vi "Param_OCVACIR.vi"(8 "errin":errorcluster, 9 "section":string="Hioki BT3562", 10 "Chaîne":string, 11 "pathin":path) -> (0 "Errout":errorcluster caption="errout", 2 "DATA":T1)   [LabVIEW 2020]
uses:
  <vilib>/Utility/config.llb/Read Key (U32).vi
  <vilib>/Utility/config.llb/Read Key (Double).vi
  <vilib>/Utility/config.llb/NI_LVConfig.lvlib
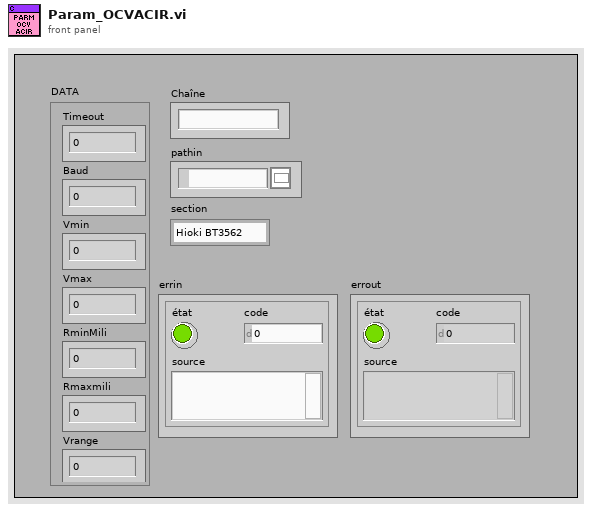
[diagram p1: front panel]
types:
  T1 = cluster{"Timeout":dbl, "Baud":u32, "Vmin":dbl, "Vmax":dbl, "RminMili":dbl, "Rmaxmili":dbl, "Vrange":dbl}
  T2 = typedef "NI_LVConfig.lvlib/Config Data RefNum.ctl" = refnum<k1>
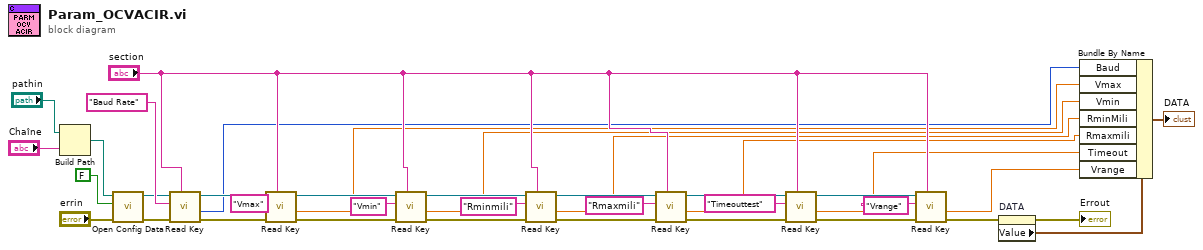
[diagram p0: block diagram]
diagram:
  n1 = Build Path(base path="pathin", name or relative path="Chaîne") -> (appended path=w18:path)
  n2 = call <vilib>:"Open Config Data.vi"("error in (no error)"="errin", "create file if necessary (T)"=FALSE, "configuration file path"=w18) -> ("error out"=w21:errorcluster, "refnum"=w17:T2)  [unwired: 6 in, 1 out]
  n3 = call-poly <vilib>:"Read Key.vi"("section"="section", "error in (no error)"=w21, "key"="Baud Rate", "refnum"=w17) -> ("error out"=w32:errorcluster, "value"=w1:u32, "refnum out"=w22:T2)  [unwired: 4 in, 1 out]
  n4 = call-poly <vilib>:"Read Key.vi"("section"="section", "error in (no error)"=w32, "key"="Vmax", "refnum"=w22) -> ("error out"=w33:errorcluster, "value"=w2:dbl, "refnum out"=w23:T2)  [unwired: 4 in, 1 out]
  n5 = call-poly <vilib>:"Read Key.vi"("section"="section", "error in (no error)"=w33, "key"="Vmin", "refnum"=w23) -> ("error out"=w34:errorcluster, "value"=w3:dbl, "refnum out"=w24:T2)  [unwired: 4 in, 1 out]
  n6 = call-poly <vilib>:"Read Key.vi"("section"="section", "error in (no error)"=w34, "key"="Rminmili", "refnum"=w24) -> ("error out"=w35:errorcluster, "value"=w4:dbl, "refnum out"=w25:T2)  [unwired: 4 in, 1 out]
  n7 = call-poly <vilib>:"Read Key.vi"("section"="section", "error in (no error)"=w35, "key"="Rmaxmili", "refnum"=w25) -> ("error out"=w36:errorcluster, "value"=w5:dbl, "refnum out"=w26:T2)  [unwired: 4 in, 1 out]
  n8 = call-poly <vilib>:"Read Key.vi"("section"="section", "error in (no error)"=w36, "key"="Timeouttest", "refnum"=w26) -> ("error out"=w12:errorcluster, "value"=w6:dbl, "refnum out"=w10:T2)  [unwired: 4 in, 1 out]
  n9 = call-poly <vilib>:"Read Key.vi"("section"="section", "error in (no error)"=w12, "key"="Vrange", "refnum"=w10) -> ("error out"=w11:errorcluster, "value"=w7:dbl)  [unwired: 4 in, 2 out]
  n10 = property on="DATA" class="Clust (strict)"(error in=w11) -> (error out=→"Errout":errorcluster, "Value"=w15:T1)  [unwired: 1 in, 1 out]
  n11 = Bundle By Name(cluster=w15, "Baud"=w1, "Vmax"=w2, "Vmin"=w3, "RminMili"=w4, "Rmaxmili"=w5, "Timeout"=w6, "Vrange"=w7) -> (→"DATA":T1)
